vi "get_attribute_int32_numeric_value.vi"(7 "Attribute":T1={"Identifier"="", "Descriptive Name"="", "Data Type"=enum."Integer 32", "Command"="", "Access"=enum."Read/Write", "Range Table"="", "Read Callback"="", "Write Callback"="", "Supported Models"="", "Instrument Options"="", "Index"=0, "OPC Wait"=FALSE, "No Status Check"=FALSE, "Cache Only"=FALSE}, 8 "error in":errorcluster caption="error in (no error)", 10 "Cmd Value in":string, 11 "VISA resource name":refnum<visa-resource-name>) -> (0 "error out":errorcluster, 2 "Int32 value out":i32, 3 "VISA resource name out":refnum<visa-resource-name>)   [LabVIEW 2020, in "Rohde&Schwarz RTx Oscilloscopes.lvlib" / "rsidr_core.lvlib"]
doc: "Use this VI to covert the instrument response to the Int32 attribute value when reading from the instrument.\nTakes the string input value and converts it to the integer value.\nFor attributes with discrete range tables the value is converted by searching for an item with the matching input string.\nOtherwise the VIs performs String->Int32 conversion using either ascii conversion or binary conversion."
uses:
  rsidr_core.lvlib
  type_Attribute.ctl
  type_Attribute_Data_Type.ctl
  type_ReadWriteAccess.ctl
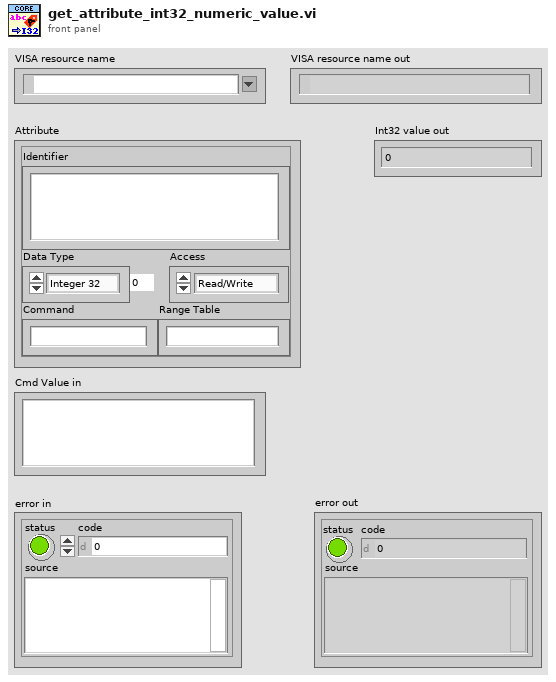
[diagram p1: front panel]
types:
  T1 = typedef "Rohde&Schwarz RTx Oscilloscopes.lvlib/rsidr_core.lvlib/type_Attribute.ctl" = cluster{"Identifier":string, "Descriptive Name":string, "Data Type":T2, "Command":string, "Access":T3, "Range Table":string, "Read Callback":string, "Write Callback":string, "Supported Models":string, "Instrument Options":string, "Index":i32, "OPC Wait":bool, "No Status Check":bool, "Cache Only":bool}
  T2 = typedef "Rohde&Schwarz RTx Oscilloscopes.lvlib/rsidr_core.lvlib/type_Attribute_Data_Type.ctl" = enum16{"Integer 32", "Double", "String", "Boolean", "None", "Integer 64", "RawString"}
  T3 = typedef "Rohde&Schwarz RTx Oscilloscopes.lvlib/rsidr_core.lvlib/type_ReadWriteAccess.ctl" = enum16{"Read Only", "Write Only", "Read/Write"}
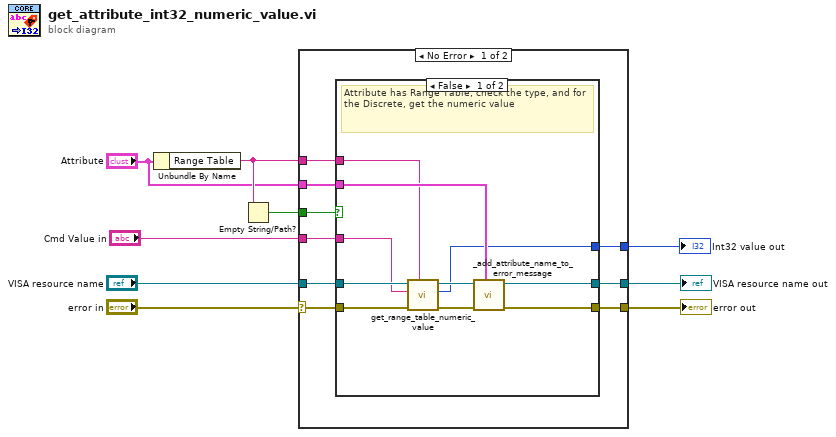
[diagram p0: block diagram]
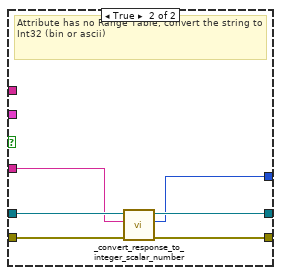
[diagram p2: hidden frame]
diagram:
  n1 = Unbundle By Name("Attribute") -> ("Range Table"=w6:string)
  n2 = Empty String/Path?(string/path=w6) -> (empty?=w7:bool)
  n3 = case shown="No Error" "error in" {
    selector: "error in" -> [w12 w36]
    tunnel: "VISA resource name" -> [w11 w35]
    tunnel: [w18 w36] -> w9
    tunnel: [w17 w35] -> w8
    tunnel: w7 -> [w16 _]
    tunnel: w6 -> [w15 _]
    tunnel: [w14 _] -> w5
    tunnel: "Cmd Value in" -> [w13 _]
    tunnel: "Attribute" -> [w10 _]
    frame No Error {
      n4 = case shown="False" w16 {
        tunnel: w12 -> [w25 w34]
        tunnel: w11 -> [w24 w33]
        tunnel: w13 -> [w21 w30]
        tunnel: [w19 w29] -> w14
        tunnel: [w28 w32] -> w18
        tunnel: [w27 w31] -> w17
        tunnel: w15 -> [w20 _]
        tunnel: w10 -> [w26 _]
        frame False {
          # "Attribute has Range Table, check the type, and for the Discrete, get the numeric value"
          n5 = call "get_range_table_numeric_value.vi"("Range Table ID in"=w20, "error in"=w25, "String Value"=w21, "VISA resource name"=w24) -> ("error out"=w23:errorcluster, "I32 output"=w19:i32, "VISA resource name out"=w22:refnum<visa-resource-name>)  [unwired: 5 in]
          n6 = call "_add_attribute_name_to_error_message.vi"("Attribute"=w26, "error in"=w23, "VISA resource name"=w22) -> ("error out"=w28:errorcluster, "VISA resource name out"=w27:refnum<visa-resource-name>)  [unwired: 6 in, 1 out]
        }
        frame True {
          # "Attribute has no Range Table, convert the string to Int32 (bin or ascii)"
          n7 = call "_convert_response_to_integer_scalar_number.vi"("error in"=w34, "Input string"=w30, "VISA resource name"=w33) -> ("error out"=w32:errorcluster, "Int32 out"=w29:i32, "VISA resource name out"=w31:refnum<visa-resource-name>)  [unwired: 6 in]
        }
      }
    }
    frame Error {
    }
  }
  "VISA resource name out" <- w8
  "error out" <- w9
  "Int32 value out" <- w5
